vi "QuitDM_STED.vi"   [LabVIEW 2014]
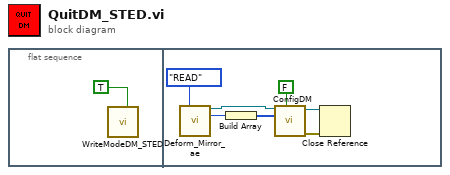
[diagram p0: block diagram]
diagram:
  n1 = flat-sequence {
    frame #0 {
      n2 = call "WriteModeDM_STED.vi"("ClearV"=TRUE) -> ()  [unwired: 9 in, 2 out]
    }
    frame #1 {
      n3 = call "Deform_Mirror_ae.vi"("Enum"=enum16{"WRITE", "READ"}."READ") -> ("Refnum Out"=w5:refnum<k7>, "IDs Out"=w3:i32)  [unwired: 10 in, 3 out]
      n4 = Build Array(w3) -> (w2:i32[])
      n5 = call "ConfigDM.vi"("High Voltage"=FALSE, "Dev IDs"=w2, "Automation Refnum in"=w5) -> ("error out"=w4:errorcluster, "Automation Refnum out"=w6:refnum<k7>)  [unwired: 7 in]
      n6 = Close Reference(reference=w6, error in (no error)=w4) -> ()  [unwired: 1 out]
    }
  }
